vi "angle_between_two_vectors.vi"(1 "B Vector":dbl[](array[numeric]), 2 "A Vector":dbl[](array[numeric])) -> (0 "degree":dbl)   [LabVIEW 2018]
doc: "This example calculates the angle between two vectors, using two different methods. The first method uses the following equation:\n Vector 1 (dot product) Vector 2\n Cosine(theta) = --------------------------------------\n ||Vector 1|| X || Vector 2 ||\n\nwhere the . (dot) is the dot product between the vectors and || Vector|| = the magnitude of the vector.\n\nA limitation of this method is that theta is between 0 and 180.\n\nThe second method uses the complex LabVIEW math routines to calculate each vector phase. To compute theta, the VI calculates the difference between the phase of each vector.\n\nA limitation of this method is that it might be 180 degrees out of phase from the first method."
uses:
  <vilib>/Analysis/_algsub.llb/Real Vector Norm.vi
  <vilib>/Analysis/baseanly.llb/Real Dot Product.vi
  <vilib>/Analysis/NI_AALPro.lvlib
  <vilib>/Analysis/NI_AALBase.lvlib
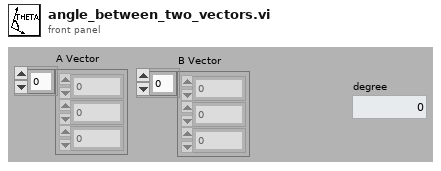
[diagram p1: front panel]
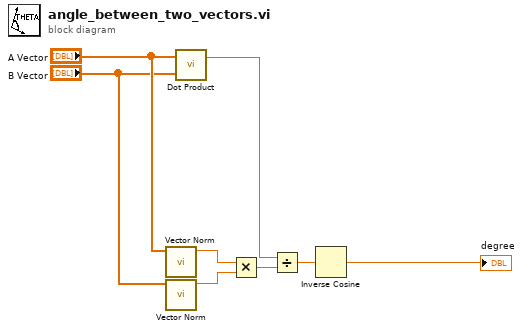
[diagram p0: block diagram]
diagram:
  n1 = call-poly <vilib>:"Vector Norm.vi"("Input Vector"="A Vector") -> ("norm"=w4:dbl)  [unwired: 9 in, 1 out]
  n2 = call-poly <vilib>:"Vector Norm.vi"("Input Vector"="B Vector") -> ("norm"=w7:dbl)  [unwired: 9 in, 1 out]
  n3 = call-poly <vilib>:"Dot Product.vi"("Y Vector"="B Vector", "X Vector"="A Vector") -> ("X * Y"=w8:dbl)  [unwired: 1 out]
  n4 = Multiply(x=w4, y=w7) -> (x*y=w6:dbl)
  n5 = Divide(x=w8, y=w6) -> (x/y=w5:dbl)
  n6 = Inverse Cosine(1:w5) -> (0:→"degree":dbl)
